vi "Menu Act.vi"(10 "LayoutMap":map{string, T1}(c390), 11 "Menu in":refnum<k9>) -> ()   [LabVIEW 2020, in "MDI ViewManager.lvlib"]
uses:
  MDI ViewManager.lvlib
  Typedef/Layout.ctl
  <vilib>/Utility/miscctls.llb/LVPointTypeDef.ctl
  <vilib>/Utility/miscctls.llb/LVBoundsTypeDef.ctl
  <vilib>/Utility/miscctls.llb/LVPositionTypeDef.ctl
  <vilib>/Utility/miscctls.llb/LVRectTypeDef.ctl
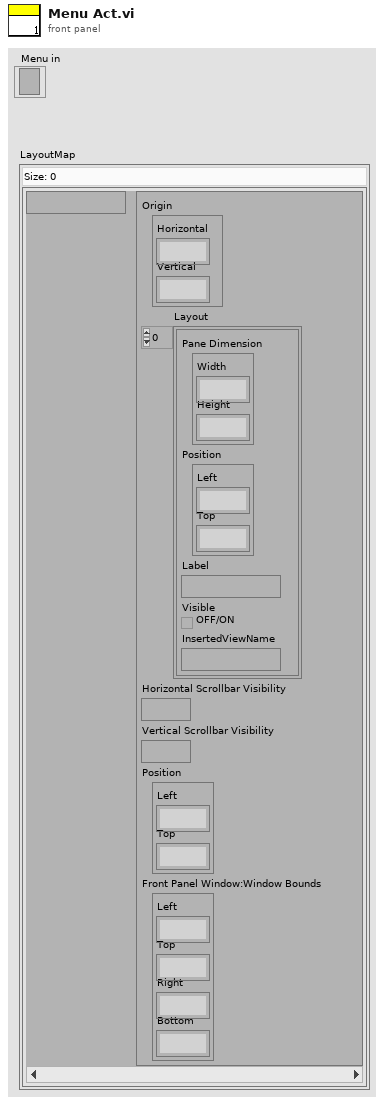
[diagram p1: front panel]
types:
  T1 = typedef "MDI ViewManager.lvlib/Layout.ctl" = cluster{"Origin":T2, "Layout":cluster{"Pane Dimension":T3, "Position":T4, "Label":string, "Visible":bool, "InsertedViewName":string}[], "Horizontal Scrollbar Visibility":enum16{"Always On", "Always Off", "Off While Running"}, "Vertical Scrollbar Visibility":enum16{"Always On", "Always Off", "Off While Running"}, "Position":T4, "Rect":T5}
  T2 = typedef "LVPointTypeDef.ctl" = cluster{"Horizontal":i16, "Vertical":i16}
  T3 = typedef "LVBoundsTypeDef.ctl" = cluster{"Width":u32, "Height":u32}
  T4 = typedef "LVPositionTypeDef.ctl" = cluster{"Left":i32, "Top":i32}
  T5 = typedef "LVRectTypeDef.ctl" = cluster{"Left":i16, "Top":i16, "Right":i16, "Bottom":i16}
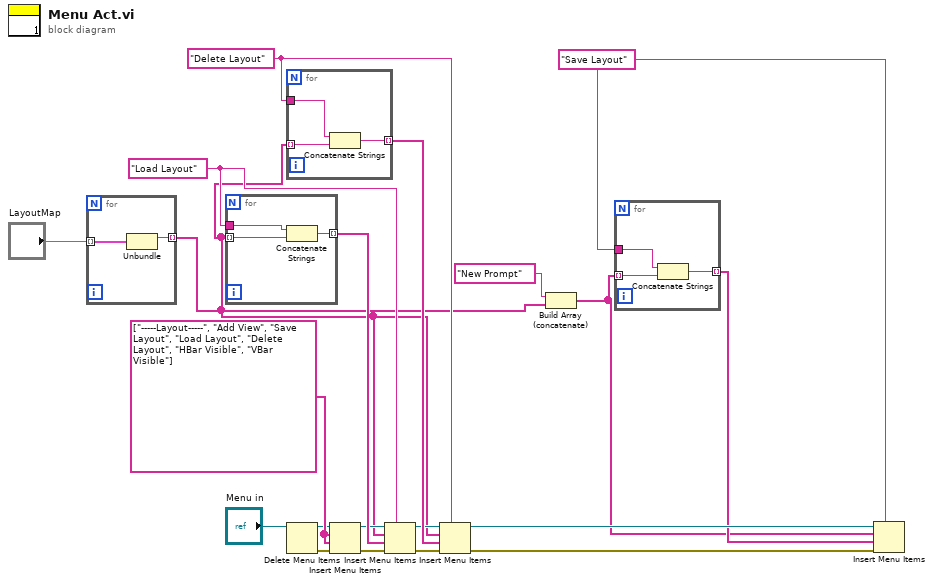
[diagram p0: block diagram]
diagram:
  w5 = "Save Layout"
  w19 = "Delete Layout"
  w17 = "Load Layout"
  w10 = string[] ["-----Layout-----", "Add View", "Save Layout", "Load Layout", "Delete Layout", "HBar Visible", "VBar Visible"] ("item names")
  n1 = for {
    tunnel: "LayoutMap" -> [w22] mode=indexing
    tunnel: [w21] -> w3 mode=indexing
    n2 = Unbundle(w22) -> (w21:string)  [unwired: 1 out]
  }
  n3 = for {
    tunnel: w3 -> [w25] mode=indexing
    tunnel: w17 -> [w24]
    tunnel: [w23] -> w18 mode=indexing
    n4 = Concatenate Strings(w24, w25) -> (w23:string)
  }
  n5 = for {
    tunnel: w3 -> [w28] mode=indexing
    tunnel: w19 -> [w27]
    tunnel: [w26] -> w20 mode=indexing
    n6 = Concatenate Strings(w27, w28) -> (w26:string)
  }
  n7 = Delete Menu Items(9:"Menu in") -> (0:w8:errorcluster, 3:w9:refnum<k9>)  [unwired: 3 in]
  n8 = Insert Menu Items(6:w8, 7:w10, 8:w10, 9:w9) -> (0:w13:errorcluster, 3:w14:refnum<k9>)  [unwired: 2 in, 1 out]
  n9 = Insert Menu Items(5:w17, 6:w13, 7:w18, 8:w3, 9:w14) -> (0:w16:errorcluster, 3:w15:refnum<k9>)  [unwired: 1 in, 1 out]
  n10 = Insert Menu Items(5:w19, 6:w16, 7:w20, 8:w3, 9:w15) -> (0:w7:errorcluster, 3:w6:refnum<k9>)  [unwired: 1 in, 1 out]
  n11 = Build Array (concatenate)("New Prompt", w3) -> (w1:string[])
  n12 = for {
    tunnel: w1 -> [w31] mode=indexing
    tunnel: w5 -> [w30]
    tunnel: [w29] -> w4 mode=indexing
    n13 = Concatenate Strings(w30, w31) -> (w29:string)
  }
  n14 = Insert Menu Items(5:w5, 6:w7, 7:w4, 8:w1, 9:w6) -> ()  [unwired: 1 in, 3 out]
